vi "macro_ElevatorFF_Calculate.vi"   [LabVIEW 2019, in "Trajectory_Library.lvlib"]
uses:
  Trajectory_Library.lvlib
types:
  T1 = typedef "Trajectory_Library.lvlib/ELEV_FF.ctl" = cluster{"Ks":dbl, "Kv":dbl, "Ka":dbl, "Kg":dbl}
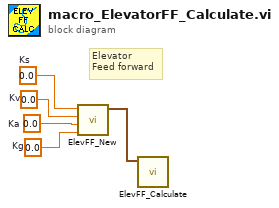
[diagram p0: block diagram]
diagram:
  w1 = 0.0  # Ks
  w2 = 0.0  # Kv
  w3 = 0.0  # Ka
  w4 = 0.0  # Kg
  # "Elevator\nFeed forward"
  n1 = call "ElevFF_New.vi"("Kg"=w4, "Ka"=w3, "Kv"=w2, "Ks"=w1) -> ("ELEV_FF"=w5:T1)  [unwired: 7 in]
  n2 = call "ElevFF_Calculate.vi"("in ELEV_FF"=w5) -> ()  [unwired: 10 in, 1 out]
